vi "Get Project References.vi"(8 "error in":errorcluster, 10 "Target Selection":string, 11 "Project in":refnum<vi>) -> (0 "error out":errorcluster, 3 "References":T1)   [LabVIEW 2019, in "Panther Dashboard.lvlib"]
uses:
  Panther Dashboard.lvlib
  Project References--cluster.ctl
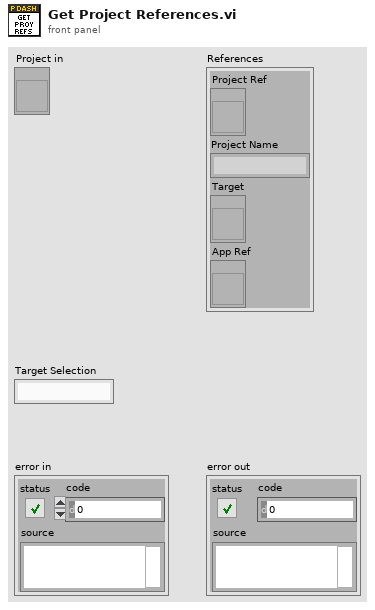
[diagram p1: front panel]
types:
  T1 = typedef "Panther Dashboard.lvlib/Project References--cluster.ctl" = cluster{"Project Ref":refnum<vi>, "Project Name":string, "Target":refnum<vi>, "App Ref":refnum<vi>}
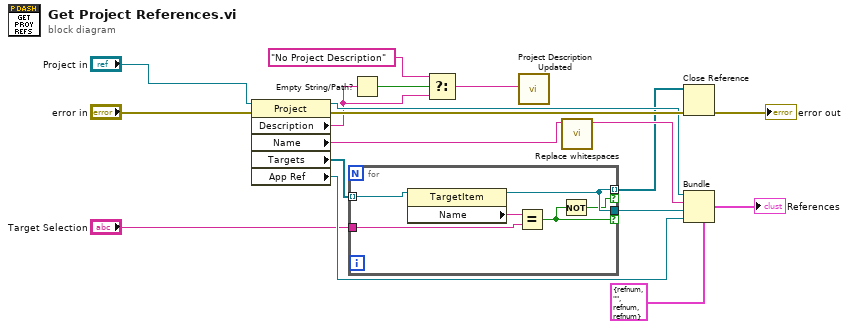
[diagram p0: block diagram]
diagram:
  n1 = property class="Project"(reference="Project in", error in="error in") -> (reference out=w15:refnum<vi>, error out=w18:errorcluster, "Description"=w12:string, "Name"=w13:string, "Targets"=w4:refnum<vi>[], "App Ref"=w7:refnum<vi>)
  n2 = for {
    tunnel: w4 -> [w24] mode=indexing
    tunnel: "Target Selection" -> [w22]
    tunnel: [w20] -> w6 if=w21
    tunnel: [w20] -> w11 mode=indexing if=w19
    n3 = property class="TargetItem"(reference=w24) -> (reference out=w20:refnum<vi>, "Name"=w23:string)  [unwired: 1 in, 1 out]
    n4 = Equal?(x=w23, y=w22) -> (x = y?=w21:bool)
    n5 = Not(x=w21) -> (.not. x?=w19:bool)
  }
  n6 = Empty String/Path?(string/path=w12) -> (empty?=w8:bool)
  n7 = Select(t="No Project Description", s=w8, f=w12) -> (s? t:f=w9:string)
  n8 = call "Project Description Updated.vi"("Project Description"=w9) -> ()  [unwired: 10 in, 1 out]
  n9 = call "Replace whitespaces.vi"("Text"=w13) -> ("text with spaces replaced"=w14:string)  [unwired: 10 in]
  n10 = Close Reference(reference=w11, error in (no error)=w18) -> (error out=→"error out":errorcluster)
  n11 = Bundle(cluster=T1 {"Project Ref"=refnum, "Project Name"="", "Target"=refnum, "App Ref"=refnum} ("References"), "Project Ref"=w15, "Project Name"=w14, "Target"=w6, "App Ref"=w7) -> (→"References":T1)
